vi "10 Encoder.vi"() -> ()   [LabVIEW 2018]
doc: "This example shows how to configure, read values from, and reset an encoder.\n\nIt will display the encoder value, period, direction, and if the encoder is stopped.\n\nThis example expects a USB cable connected from your development PC to the Type B USB Jack (next to the power input) on the roboRIO."
uses:
  <vilib>/Rock Robotics/SystemInterfaces/DIO/FPGA_DIOChannel.ctl
  <vilib>/Rock Robotics/WPI/Encoder/WPI_EncoderType.ctl
  <vilib>/Rock Robotics/WPI/Counter/WPI_CounterDigitalInputToDigitalSource.vi
panel:
  in  "Number Samples to Average":u8=1 min=1 max=128
  in  "Invert Direction":bool
  in  "Decoding Type":T1=enum."4x"
  in  "DistancePerCount":dbl=1.0
  in  "B Channel":T2=enum."DIO 3"
  in  "A Channel":T2=enum."DIO 2"
  out "Encoder Rate (distance/sec)":dbl
  out "Encoder Distance":dbl
  in  "Minimum Rate":dbl=20.0
  in  "stop":bool
  in  "Reset Encoder?":bool
  out "Encoder Alarm Status":string
  out "Encoder Direction":string
  # "Set these inputs before running."
  # "This can be set while running."
  # "Output information."
  # "This shows wiring for a generic quadrature encoder.  Some encoders may have Gnd labeled as Com.  Some may have +5V labeled as +VDC."
  # "Encoder\nB (white wire)---------\nGnd (black wire)------\n+5V (red wire)---------\nA (white wire)---------"
  # "roboRIO\nDIO-1  S\nDIO-0 \nDIO-0  V\nDIO-0  S"
  # "Encoder"
  # "Index"
  # "Gnd"
  # "+5V"
  # "B"
  # "A"
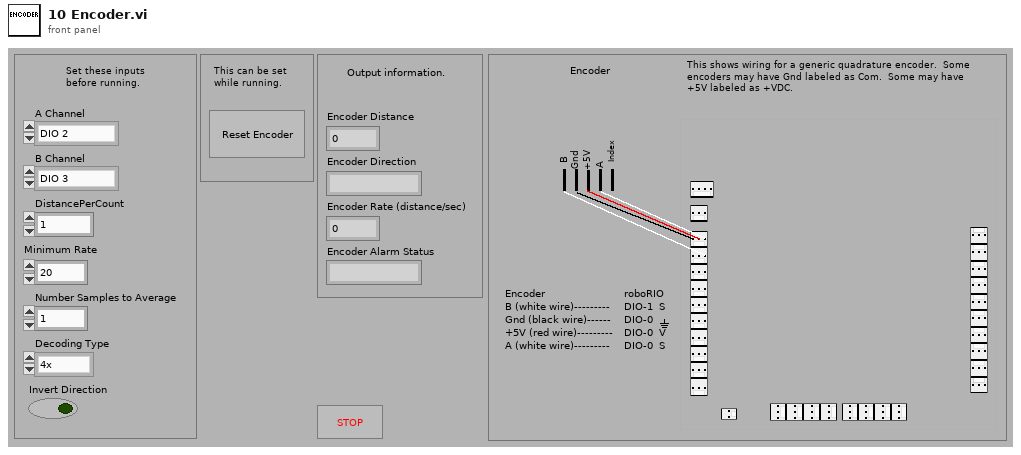
[diagram p1: front panel]
types:
  T1 = typedef "WPI_EncoderType.ctl" = enum16{"1x", "2x", "4x"}
  T2 = typedef "FPGA_DIOChannel.ctl" = enum8{"DIO 0", "DIO 1", "DIO 2", "DIO 3", "DIO 4", "DIO 5", "DIO 6", "DIO 7", "DIO 8", "DIO 9", "DIO MXP 0", "DIO MXP 1", "DIO MXP 2", "DIO MXP 3", "DIO MXP 4", "DIO MXP 5", "DIO MXP 6", "DIO MXP 7", "DIO MXP 8", "DIO MXP 9", "DIO MXP 10", "DIO MXP 11", "DIO MXP 12", "DIO MXP 13", "DIO MXP 14", "DIO MXP 15", "SPI Port CS1", "SPI Port CS2", "SPI Port CS3", "SPI Port MISO", "SPI Port MOSI", "Invalid"}
  T3 = typedef "WPI_DigitalInputDevRef.ctl" = cluster{"DevStatus":errorcluster, "DIO Channel":T2}
  T4 = typedef "FPGA_CounterEncoderSourceConvertionLVSourceType.ctl" = cluster{"DevStatus":errorcluster, "AnalogTriggerMode?":bool, "DigitalMode":cluster{"DIO Channel":T5}, "AnalogTriggerMode":cluster{"AnalogTriggerIndex":T6, "OutputType":T7}}
  T5 = typedef "FPGA_DIODigitalSourceChannel.ctl" = enum8{"DIO 0", "DIO 1", "DIO 2", "DIO 3", "DIO 4", "DIO 5", "DIO 6", "DIO 7", "DIO 8", "DIO 9", "DIO MXP 0", "DIO MXP 1", "DIO MXP 2", "DIO MXP 3", "DIO MXP 4", "DIO MXP 5", "DIO MXP 6", "DIO MXP 7", "DIO MXP 8", "DIO MXP 9", "DIO MXP 10", "DIO MXP 11", "DIO MXP 12", "DIO MXP 13", "DIO MXP 14", "DIO MXP 15", "SPI Port CS1", "SPI Port CS2", "SPI Port CS3", "SPI Port MISO", "SPI Port MOSI", "Disabled"}
  T6 = typedef "FPGA_AnalogTriggerIndex.ctl" = enum8{"Trig 0", "Trig 1", "Trig 2", "Trig 3", "Trig 4", "Trig 5", "Trig 6", "Trig 7", "Invalid"}
  T7 = typedef "FPGA_AnalogTriggerOutType.ctl" = enum16{"InWindow", "TriggerState", "Rising", "Falling"}
  T8 = typedef "WPI_EncoderDevRef.ctl" = cluster{"DevStatus":errorcluster, "EncoderIndex":T9, "CounterIndex":T10, "DistancePerCount":dbl, "Decoding Type":T1}
  T9 = typedef "FPGA_EncoderIdx.ctl" = enum8{"Enc 0", "Enc 1", "Enc 2", "Enc 3", "Enc 4", "Enc 5", "Enc 6", "Enc 7", "Invalid"}
  T10 = typedef "FPGA_CounterCtrSystemIndex.ctl" = enum8{"Ctr 0", "Ctr 1", "Ctr 2", "Ctr 3", "Ctr 4", "Ctr 5", "Ctr 6", "Ctr 7", "Invalid"}
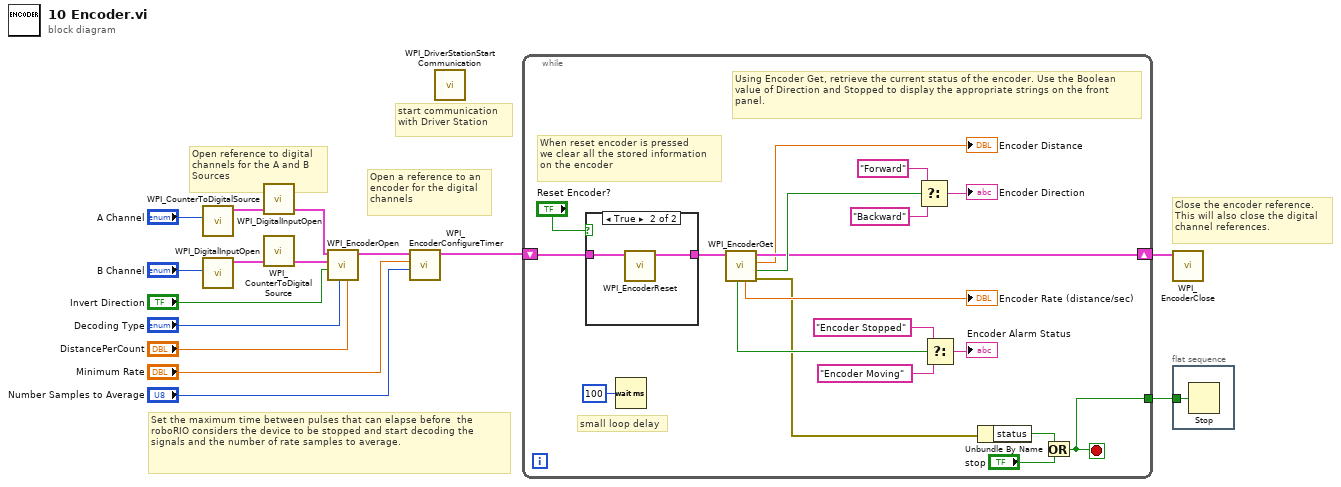
[diagram p0: block diagram]
diagram:
  # "start communication with Driver Station"
  # "Close the encoder reference.\nThis will also close the digital \nchannel references."
  # "Set the maximum time between pulses that can elapse before  the roboRIO considers the device to be stopped and start decoding the signals and the number of rate samples to average."
  # "Open a reference to an\nencoder for the digital \nchannels"
  # "Open reference to digital \nchannels for the A and B\nSources"
  n1 = call <vilib>:"WPI_DigitalInputOpen.vi"("DIO Channel"="A Channel") -> ("DigitalInputDevRef"=w12:T3)  [unwired: 1 in, 9 out]
  n2 = call <vilib>:"WPI_DigitalInputOpen.vi"("DIO Channel"="B Channel") -> ("DigitalInputDevRef"=w13:T3)  [unwired: 1 in, 9 out]
  n3 = call-poly <vilib>:"WPI_CounterToDigitalSource.vi"("DigitalInputDevRef"=w12) -> ("Digital Source"=w11:T4)  [unwired: 6 out]
  n4 = call-poly <vilib>:"WPI_CounterToDigitalSource.vi"("DigitalInputDevRef"=w13) -> ("Digital Source"=w14:T4)  [unwired: 6 out]
  n5 = call <vilib>:"WPI_EncoderOpen.vi"("DistancePerCount"="DistancePerCount", "Decoding Type"="Decoding Type", "Invert Direction (False)"="Invert Direction", "BSource"=w14, "ASource"=w11) -> ("EncoderDevRef"=w4:T8)  [unwired: 3 in, 3 out]
  n6 = call <vilib>:"WPI_EncoderConfigureTimer.vi"("Number Samples to Average"="Number Samples to Average", "Minimum Rate"="Minimum Rate", "EncoderDevRef"=w4) -> ("EncoderDevRef"=w5:T8)  [unwired: 1 in, 7 out]
  n7 = call <vilib>:"WPI_DriverStationStart Communication.vi"() -> ()  [unwired: 2 in, 10 out]
  n8 = while {
    shift-right: [w27] -> w15
    shift-left: w5 -> [w32]
    tunnel: [w24] -> w1
    stop <- w24 stop-if-true
    # "small loop delay"
    # "Using Encoder Get, retrieve the current status of the encoder. Use the Boolean value of Direction and Stopped to display the appropriate strings on the front panel."
    # "When reset encoder is pressed\nwe clear all the stored information\non the encoder"
    n9 = case shown="True" "Reset Encoder?" {
      tunnel: w32 -> [w35 w37]
      tunnel: [w35 w36] -> w30
      frame False {
      }
      frame True {
        n10 = call <vilib>:"WPI_EncoderReset.vi"("EncoderDevRef"=w37) -> ("EncoderDevRef"=w36:T8)  [unwired: 1 in, 9 out]
      }
    }
    n11 = Wait (ms)(milliseconds to wait=u32 100) -> ()  [unwired: 1 out]
    n12 = call <vilib>:"WPI_EncoderGet.vi"("EncoderDevRef"=w30) -> ("error out"=w22:errorcluster, "Direction"=w29:bool, "Distance"=→"Encoder Distance":dbl, "EncoderDevRef"=w27:T8, "Rate"=→"Encoder Rate (distance/sec)":dbl, "Stopped"=w28:bool)  [unwired: 1 in, 4 out]
    n13 = Select(t="Forward", s=w29, f="Backward") -> (s? t:f=→"Encoder Direction":string)
    n14 = Select(t="Encoder Stopped", s=w28, f="Encoder Moving") -> (s? t:f=→"Encoder Alarm Status":string)
    n15 = Unbundle By Name(w22) -> ("status"=w20:bool)
    n16 = Or(x=w20, y="stop") -> (x .or. y?=w24:bool)
  }
  n17 = call <vilib>:"WPI_EncoderClose.vi"("EncoderDevRef"=w15) -> ()  [unwired: 2 in, 9 out]
  n18 = flat-sequence {
    tunnel: w1 -> [w38]
    frame #0 {
      n19 = Stop(stop? (T)=w38) -> ()
    }
  }
